vi "Auto Set Intake Position.vi"(10 "Intake Position":dbl, 11 "Run?":bool) -> (3 "Done":bool)   [LabVIEW 2013]
uses:
  Globals/Auto.vi
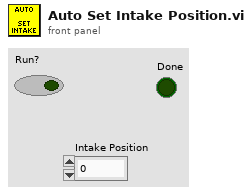
[diagram p1: front panel]
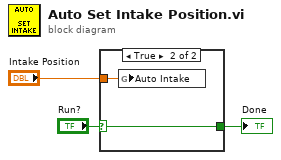
[diagram p0: block diagram]
diagram:
  n1 = case shown="True" "Run?" {
    selector: "Run?" -> [w4 w6]
    tunnel: [w4 w6] -> w2
    tunnel: "Intake Position" -> [_ w5]
    frame False {
    }
    frame True {
      n2 = global write "Auto.vi" "Auto Intake"(w5) -> ()
    }
  }
  "Done" <- w2
